vi "TDMSVisu.vi"(4 "error in (no error)":errorcluster caption="entrée d'erreur (pas d'erreur)", 7 "file path":path caption="chemin du fichier") -> (0 "error out":errorcluster caption="sortie d'erreur", 3 "file path out":path caption="chemin du fichier en sortie")   [LabVIEW 2017]
doc: "Ouvre le fichier .tdms spécifié dans l'entrée <B>chemin du fichier</B> et présente les données du fichier dans la boîte de dialogue TDMS - Afficheur de fichier."
uses:
  <vilib>/Utility/tdmsutil.llb/fileViewerConfigData.ctl
  <vilib>/Utility/error.llb/DialogType.ctl
  <vilib>/Utility/tdmsutil.llb/TDMSFileViewerLocalizedText.vi
  Instance           1 26Saved   TDMS - File Viewer .vi
panel:
  in  "Quit":bool caption="Quitter"
  in  "Properties / Values / Graph":T1(tab) caption="Propriétés / Valeurs / Graphe"
  in  "Properties":i32(listbox) caption="Propriétés"
  in  "Status":string caption="État"
  in  "Settings...":bool caption="Paramètres..."
  in  "Raw data values":i32(listbox) caption="Valeurs des données brutes"
  out "Waveform Graph":waveform(dbl)[](graph) caption="Graphe"
  in  "Help":bool caption="Aide"
  in  "File contents":string(tree) caption="Contenu du fichier"
  # "Affichage des valeurs 1..1000"
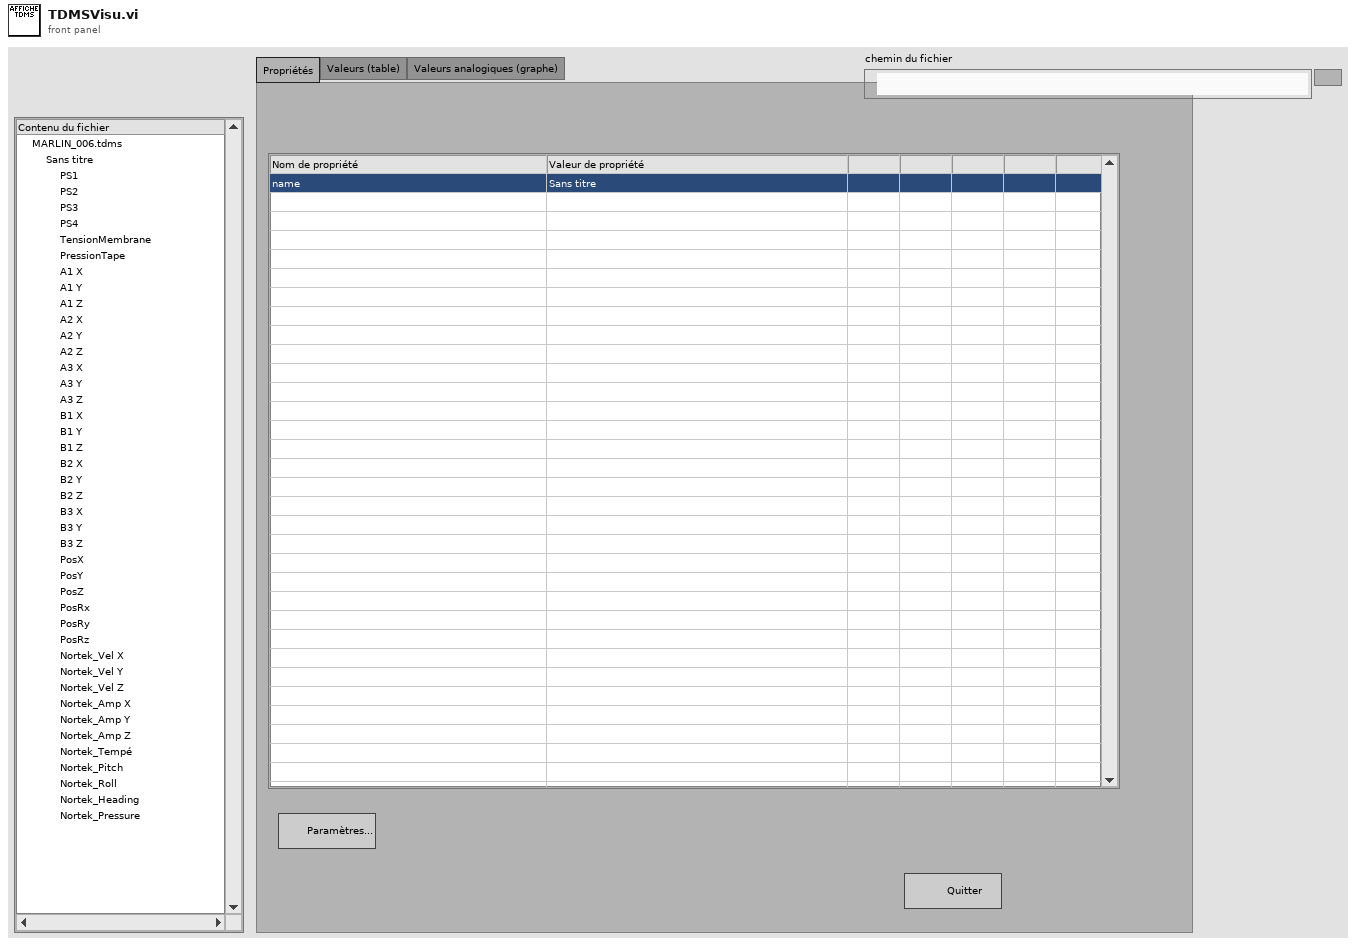
[diagram p1: front panel]
types:
  T1 = enum32{"Properties", "Values (table)", "Analog values (graph)"}
  T2 = enum16{"open", "open or create", "create or replace", "create", "open (read-only)"}
  T3 = typedef "fileViewerConfigData.ctl" = cluster{"Show all (table)":bool, "Show all (graph)":bool, "limit (table)":u64, "limit (graph)":u64, "no show":bool, "start (table)":u64, "start (graph)":u64}
  T4 = cluster{"Tree":refnum<vi>, "Tab Control":refnum<vi>, "property list":refnum<vi>, "raw data list":refnum<vi>, "Waveform Graph":refnum<vi>, "Ok":refnum<vi>, "Ok 2":refnum<vi>, "Ok 3":refnum<vi>, "Ok 4":refnum<vi>}
  T5 = typedef "DialogType.ctl" = u16
  T6 = typedef "LVRectTypeDef.ctl" = cluster{"Left":i16, "Top":i16, "Right":i16, "Bottom":i16}
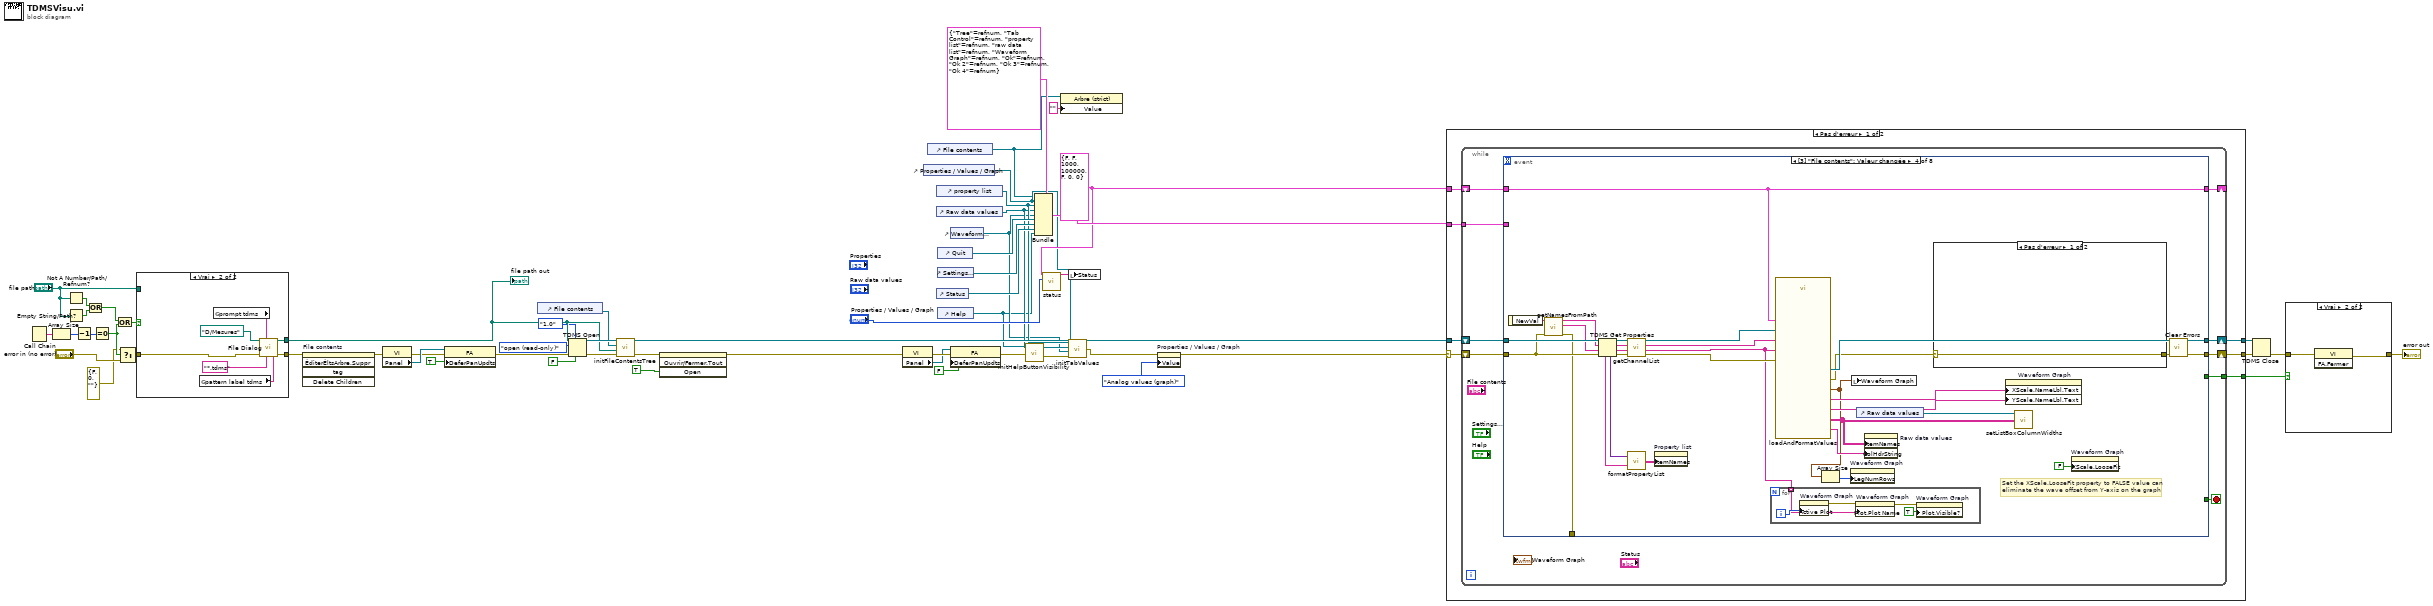
[diagram p0: block diagram]
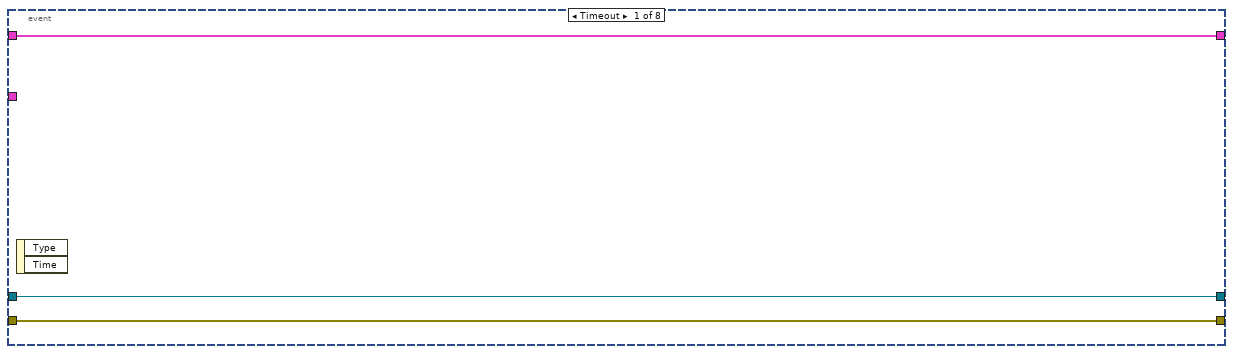
[diagram p3: hidden frame]
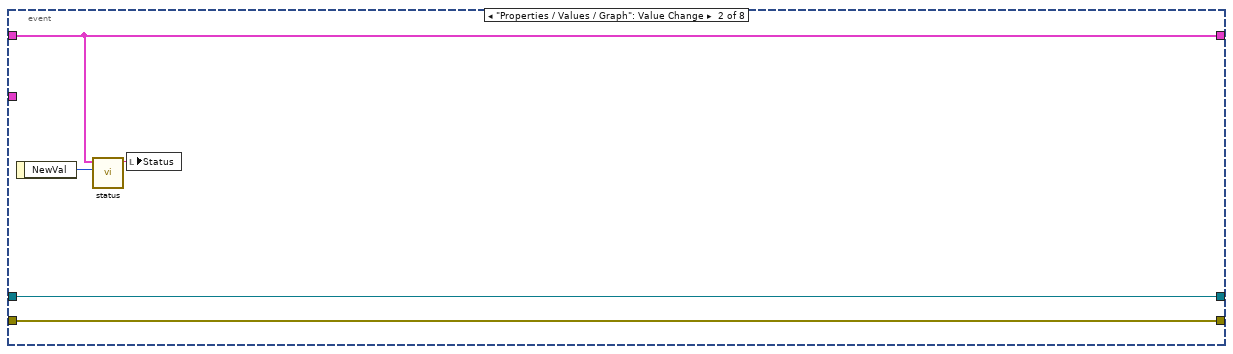
[diagram p4: hidden frame]
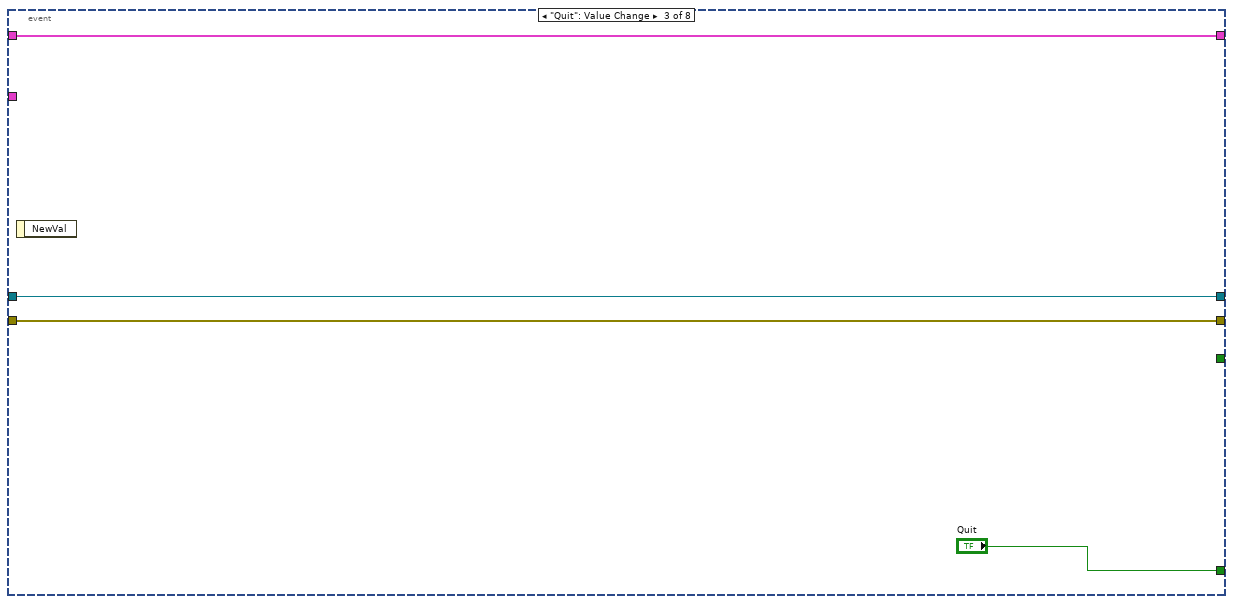
[diagram p5: hidden frame]
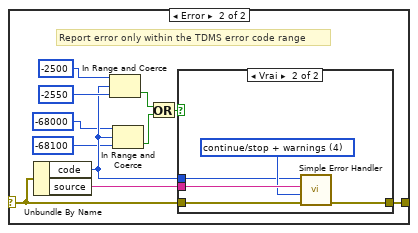
[diagram p6: hidden frame]
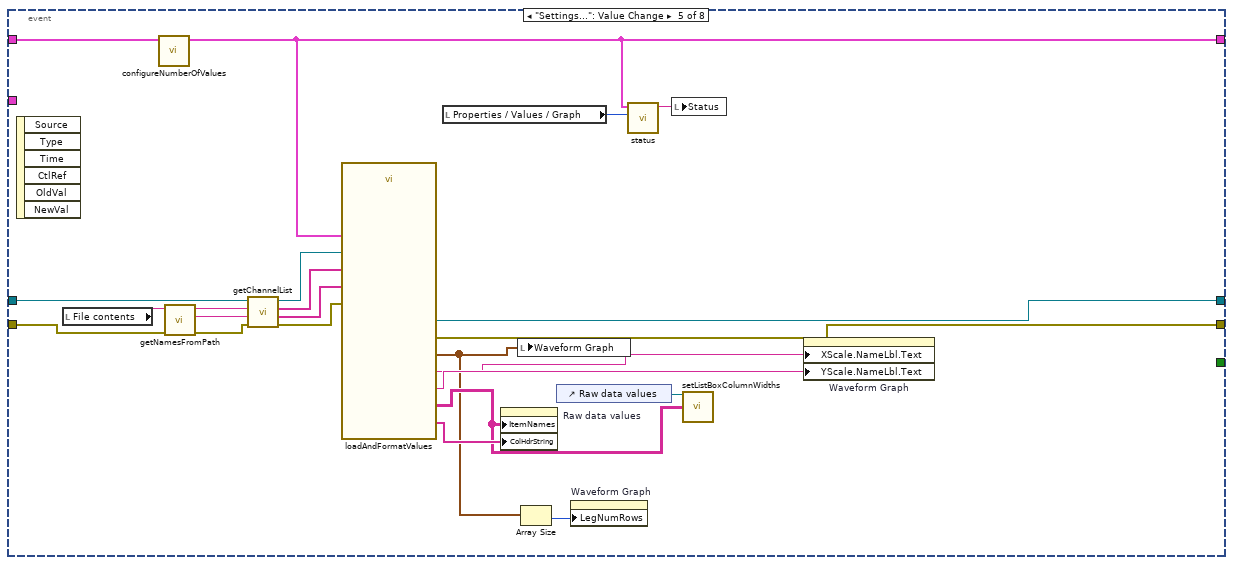
[diagram p8: hidden frame]
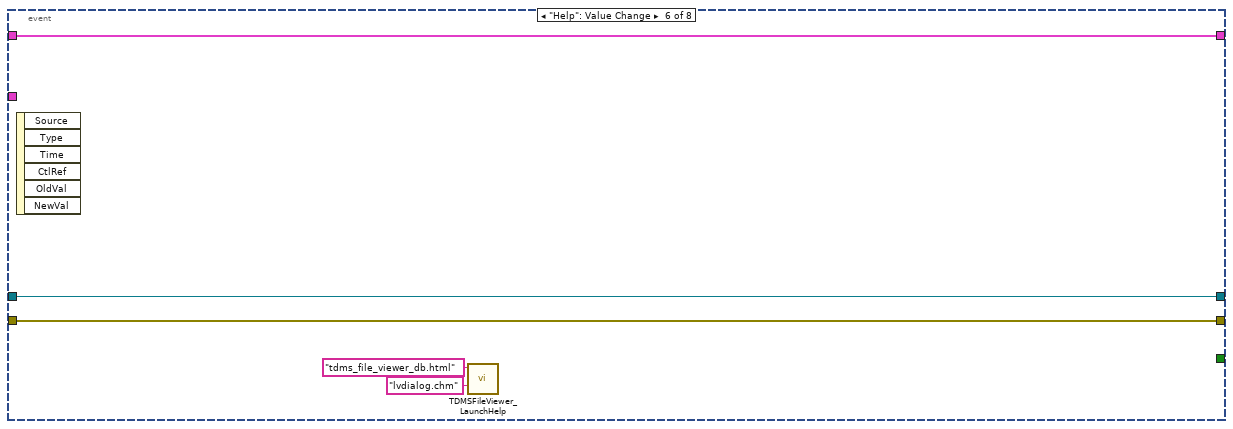
[diagram p9: hidden frame]
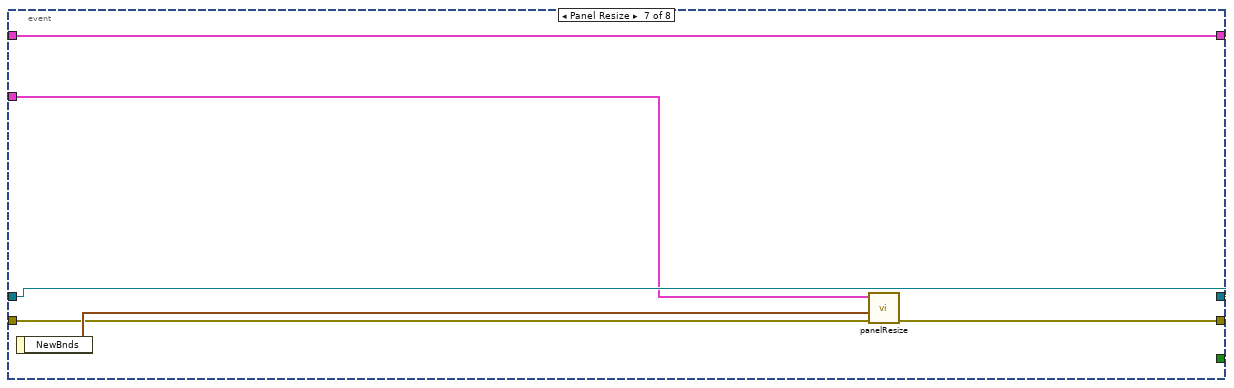
[diagram p10: hidden frame]
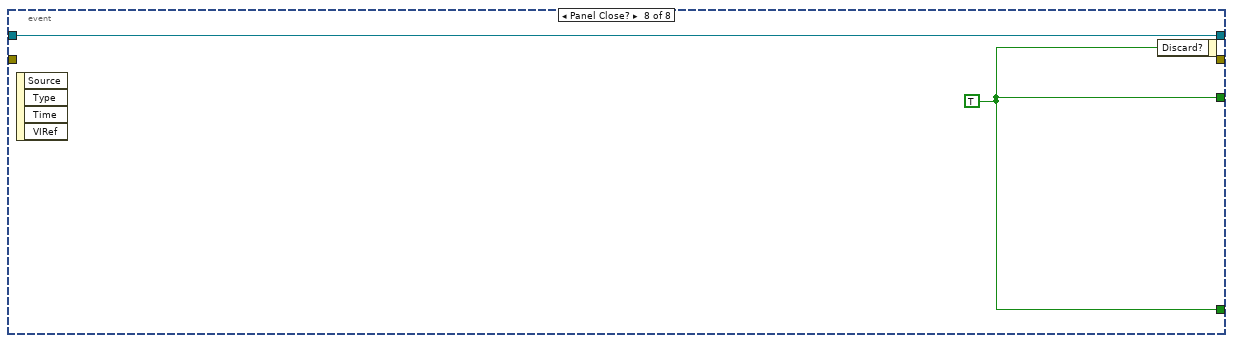
[diagram p11: hidden frame]
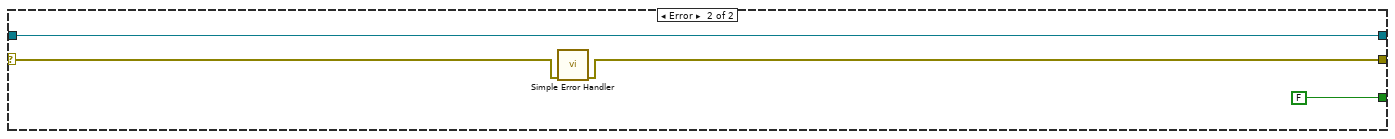
[diagram p12: hidden frame]
diagram:
  w24 = T3 {"Show all (table)"=FALSE, "Show all (graph)"=FALSE, "limit (table)"=1000, "limit (graph)"=100000, "no show"=FALSE, "start (table)"=0, "start (graph)"=0} ("TDMS File Viewer Configuration")
  n1 = Call Chain() -> (call chain=w39:string[])
  n2 = Array Size(array=w39) -> (size(s)=w37:i32)
  n3 = Not A Number/Path/Refnum?(number/path/refnum="file path") -> (NaN/Path/Refnum?=w41:bool)
  n4 = Empty String/Path?(string/path="file path") -> (empty?=w40:bool)
  n5 = Decrement(x=w37) -> (x-1=w36:i32)
  n6 = Or(x=w41, y=w40) -> (x .or. y?=w38:bool)
  n7 = Equal To 0?(x=w36) -> (x = 0?=w22:bool)
  n8 = Or(x=w38, y=w22) -> (x .or. y?=w35:bool)
  n9 = Select(t=errorcluster {"status"=FALSE, "code"=0, "source"=""}, s=w22, f="error in (no error)") -> (s? t:f=w21:errorcluster)
  n10 = case shown="Vrai" w35 {
    tunnel: [w59 w66] -> w28
    tunnel: "file path" -> [w59 _]
    tunnel: [w58 w64] -> w27
    tunnel: w21 -> [w58 w61]
    frame False {
    }
    frame True {
      n11 = global read "TDMSFileViewerLocalizedText.vi" "pattern label tdms"() -> (w62:string)
      n12 = global read "TDMSFileViewerLocalizedText.vi" "prompt tdms"() -> (w63:string)
      n13 = call "File Dialog"("start path"=path "D:/Mesures", "prompt"=w63, "error in"=w61, "pattern (all files)"="*.tdms", "pattern label"=w62) -> ("selected path"=w66:path, "error out"=w64:errorcluster)  [unwired: 2 in, 7 out]
    }
  }
  "file path out" <- w28
  n14 = invoke on="File contents" class="Tree (strict)" method="ÉditerÉltsArbre.Suppr"(error in=w27) -> (error out=w48:errorcluster)  [unwired: 4 in, 4 out]
  n15 = property class="VI"(error in=w48) -> (error out=w49:errorcluster, "Panel"=w50:refnum<vi>)  [unwired: 1 in, 1 out]
  n16 = property class="FA"(reference=w50, error in=w49, "DeferPanUpdts"=TRUE ("Defer Panel Updates")) -> (error out=w52:errorcluster)  [unwired: 1 out]
  n17 = control-ref of="File contents"() -> (w29:refnum<vi>)
  n18 = TDMS Open(6:FALSE ("disable buffering (T)"), 7:enum16{"1.0", "2.0"}."1.0" ("file format version (2.0)"), 8:w52, 10:T2."open (read-only)" ("operation"), 11:w28) -> (0:w57:errorcluster, 3:w56:refnum<k34>)  [unwired: 2 in]
  n19 = call <vilib>:"initFileContentsTree.vi"("error in (no error)"=w57, "file path"=w28, "Tree Refnum"=w29, "tdms file"=w56) -> ("error out"=w44:errorcluster, "tdms file out"=w55:refnum<k34>)  [unwired: 2 out]
  n20 = invoke on="File contents" class="Tree (strict)" method="Ouvrir/Fermer.Tout"(error in=w44, "Open"=TRUE ("Open?")) -> (error out=w3:errorcluster)  [unwired: 2 in, 3 out]
  n21 = property class="VI"(error in=w3) -> (error out=w46:errorcluster, "Panel"=w45:refnum<vi>)  [unwired: 1 in, 1 out]
  n22 = control-ref of="Properties / Values / Graph"() -> (w10:refnum<vi>)
  n23 = control-ref of="File contents"() -> (w9:refnum<vi>)
  n24 = control-ref of="property list"() -> (w13:refnum<vi>)
  n25 = control-ref of="Raw data values"() -> (w12:refnum<vi>)
  n26 = control-ref of="Status"() -> (w26:refnum<vi>)
  n27 = control-ref of="Quit"() -> (w33:refnum<vi>)
  n28 = control-ref of="Settings..."() -> (w31:refnum<vi>)
  n29 = control-ref of="Help"() -> (w5:refnum<vi>)
  n30 = control-ref of="Waveform Graph"() -> (w11:refnum<vi>)
  n31 = property class="FA"(reference=w45, error in=w46, "DeferPanUpdts"=FALSE ("Defer Panel Updates")) -> (error out=w7:errorcluster)  [unwired: 1 out]
  n32 = call <vilib>:"initHelpButtonVisibility.vi"("error in"=w7, "Help"=w5) -> ("error out"=w6:errorcluster)  [unwired: 9 in]
  n33 = Bundle(cluster=T4 {"Tree"=refnum, "Tab Control"=refnum, "property list"=refnum, "raw data list"=refnum, "Waveform Graph"=refnum, "Ok"=refnum, "Ok 2"=refnum, "Ok 3"=refnum, "Ok 4"=refnum} ("control refs"), "Tree"=w9, "Tab Control"=w10, "property list"=w13, "raw data list"=w12, "Waveform Graph"=w11, "Ok"=w33, "Ok 2"=w31, "Ok 3"=w26, "Ok 4"=w5) -> (w34:T4)
  n34 = call <vilib>:"status.vi"("tab sheet"="Properties / Values / Graph", "TDMS File Viewer Configuration"=w24) -> ("status"=w25:string)  [unwired: 5 out]
  n35 = property class="Arbre (strict)"(reference=w9, "Value"="") -> ()  [unwired: 1 in, 2 out]
  n36 = local write "Status"(w25) -> ()
  n37 = call <vilib>:"initTabValues.vi"("properties"=w13, "Values"=w12, "waveform"=w11, "error in"=w6, "Properties / Values / Graph"=w10) -> ("error out"=w2:errorcluster)
  n38 = property on="Properties / Values / Graph" class="Onglet (strict)"(error in=w2, "Value"=T1."Analog values (graph)" ("Properties / Values / Graph")) -> (error out=w1:errorcluster)  [unwired: 1 in, 1 out]
  n39 = case shown="Pas d'erreur" w1 {
    selector: w1 -> [w68 w186]
    tunnel: w55 -> [w73 w187]
    tunnel: [w72 w187] -> w54
    tunnel: [w71 w185] -> w53
    tunnel: w34 -> [w70 _]
    tunnel: w24 -> [w69 _]
    tunnel: [w67 FALSE] -> w18
    frame No Error {
      n40 = while {
        shift-right: [w80] -> w71
        shift-left: w68 -> [w81]
        shift-right: [w79] -> w72
        shift-left: w73 -> [w82]
        tunnel: w70 -> [w77]
        shift-right: [w75] -> _
        shift-left: w69 -> [w76]
        tunnel: [w74] -> w67
        stop <- w78 stop-if-true
        n41 = event shown="[3] \"File contents\": Valeur changée" {
          selector: _ -> [_ _ _ _ _ _ _ _]
          dyn-events: _ -> [_ _ _ _ _ _ _ _]
          timeout: _ -> [_ _ _ _ _ _ _ _]
          tunnel: w82 -> [w84 w89 w93 w124 w160 w174 w181 w183]
          tunnel: w81 -> [w85 w90 w92 w116 w167 w173 w178 _]
          tunnel: [w85 w90 w92 w112 w168 w173 w177 _] -> w80
          tunnel: [w84 w89 w93 w123 w169 w174 w181 w183] -> w79
          tunnel: [_ _ "Quit" _ _ _ _ w182] -> w78
          tunnel: [_ _ _ w115 _ _ _ _] -> _
          tunnel: w77 -> [_ _ _ _ _ _ w179 _]
          tunnel: w76 -> [w83 w86 w91 w105 w170 w175 w176 _]
          tunnel: [w83 w86 w91 w105 w150 w175 w176 _] -> w75
          tunnel: [_ _ _ _ _ _ _ w182] -> w74
          event Timeout {
            n42 = event-data() -> ()  [unwired: 3 out]
          }
          event "Properties / Values / Graph": Value Change {
            n43 = event-data() -> ("NewVal"=w88:T1)  [unwired: 1 out]
            n44 = call <vilib>:"status.vi"("tab sheet"=w88, "TDMS File Viewer Configuration"=w86) -> ("status"=w87:string)  [unwired: 5 out]
            n45 = local write "Status"(w87) -> ()
          }
          event "Quit": Value Change {
            n46 = event-data() -> ()  [unwired: 2 out]
          }
          event "File contents": Value Change {
            # "Set the XScale.LooseFit property to FALSE value can \neliminate the wave offset from Y-axis on the graph"
            n47 = event-data() -> ("NewVal"=w118:string)  [unwired: 1 out]
            n48 = call <vilib>:"getNamesFromPath.vi"("error in (no error)"=w116, "tree path"=w118) -> ("error out"=w115:errorcluster, "channel"=w121:string, "group"=w122:string)  [unwired: 3 out]
            n49 = TDMS Get Properties(8:w116, 9:w121, 10:w122, 11:w124) -> (0:w110:errorcluster, 1:w109:string, 2:w104:string, 3:w111:refnum<k34>, 4:w119:variant[], 6:w120:string[])  [unwired: 2 out]
            n50 = call <vilib>:"getChannelList.vi"("error in (no error)"=w110, "channel names"=w109, "group name"=w104, "tdms file"=w111) -> ("error out"=w101:errorcluster, "channel names out"=w95:string[], "group names out"=w102:string[], "tdms file out"=w103:refnum<k34>)
            n51 = call <vilib>:"formatPropertyList.vi"("property names"=w120, "property values"=w119) -> ("strings"=w117:string[][])
            n52 = property on="Property list" class="ListeMCol (strict)"("ItemNames"=w117) -> ()  [unwired: 2 in, 2 out]
            n53 = for {
              tunnel: w95 -> [w128] mode=indexing
              i -> [w129]
              n54 = property on="Waveform Graph" class="GraphWF (strict)"("Active Plot"=w129) -> (error out=w127:errorcluster)  [unwired: 2 in, 1 out]
              n55 = property on="Waveform Graph" class="GraphWF (strict)"(error in=w127, "Plot.Plot Name"=w128) -> (error out=w125:errorcluster)  [unwired: 1 in, 1 out]
              n56 = property on="Waveform Graph" class="GraphWF (strict)"(error in=w125, "Plot.Visible?"=TRUE ("Tracé.Visibles")) -> ()  [unwired: 1 in, 2 out]
            }
            n57 = call <vilib>:"loadAndFormatValues.vi"("error in (no error)"=w101, "configuration"=w105, "channel names"=w95, "group names"=w102, "tdms file"=w103) -> ("error out"=w100:errorcluster, "graph y names"=w107:string, "graph x names"=w106:string, "tdms file out"=w123:refnum<k34>, "waveform values"=w97:waveform(dbl)[], "table values"=w114:string[][], "table headers"=w108:string[])
            n58 = Array Size(array=w97) -> (size(s)=w96:i32)
            n59 = property on="Waveform Graph" class="GraphWF (strict)"("LegNumRows"=w96) -> ()  [unwired: 2 in, 2 out]
            n60 = local write "Waveform Graph"(w97) -> ()
            n61 = control-ref of="Raw data values"() -> (w113:refnum<vi>)
            n62 = property on="Raw data values" class="ListeMCol (strict)"("ItemNames"=w114, "ColHdrString"=w108) -> ()  [unwired: 2 in, 2 out]
            n63 = case shown="Pas d'erreur" w100 {
              selector: w100 -> [w130 w140]
              tunnel: [w130 w139] -> w99
              frame No Error {
              }
              frame Error {
                # "Report error only within the TDMS error code range"
                n64 = Unbundle By Name(w140) -> ("code"=w136:i32, "source"=w141:string)
                n65 = In Range and Coerce(upper limit=-2500, x=w136, lower limit=-2550 ("upper limit")) -> (In Range?=w133:bool)  [unwired: 1 out]
                n66 = In Range and Coerce(upper limit=-68000, x=w136, lower limit=-68100) -> (In Range?=w132:bool)  [unwired: 1 out]
                n67 = Or(x=w133, y=w132) -> (x .or. y?=w131:bool)
                n68 = case shown="Vrai" w131 {
                  tunnel: w141 -> [_ w147]
                  tunnel: w140 -> [w142 w146]
                  tunnel: [w142 w145] -> w139
                  tunnel: w136 -> [_ w143]
                  frame False {
                    # "Out of the range of TDMS\nerror code, we don't report\nthem."
                  }
                  frame True {
                    w144 = T5 4 items=["no dialog", "OK message", "continue or stop message", "OK message + warnings", "continue/stop + warnings"] ("type of dialog (OK msg:1)")
                    n69 = call <vilib>:"Simple Error Handler.vi"("error code (no error:0)"=w143, "error source (\" \")"=w147, "type of dialog (OK msg:1)"=w144, "error in (no error)"=w146) -> ("error out"=w145:errorcluster)  [unwired: 1 in, 4 out]
                  }
                }
              }
            }
            n70 = property on="Waveform Graph" class="GraphWF (strict)"("XScale.NameLbl.Text"=w106, "YScale.NameLbl.Text"=w107) -> ()  [unwired: 2 in, 2 out]
            n71 = call <vilib>:"setListBoxColumnWidths.vi"("table data"=w114, "MCListbox Refnum"=w113) -> ()  [unwired: 1 out]
            n72 = property on="Waveform Graph" class="GraphWF (strict)"("XScale.LooseFit"=FALSE ("X Scale.Loose Fit")) -> ()  [unwired: 2 in, 2 out]
            n73 = call <vilib>:"Clear Errors.vi"("error in (no error)"=w99) -> ("error out"=w112:errorcluster)  [unwired: 1 in, 5 out]
          }
          event "Settings...": Value Change {
            n74 = event-data() -> ()  [unwired: 7 out]
            n75 = local read "File contents"() -> (w161:string)
            n76 = call <vilib>:"configureNumberOfValues.vi"("TDMS File Viewer Configuration"=w170) -> ("TDMS File Viewer Configuration Out"=w150:T3)  [unwired: 10 out]
            n77 = call <vilib>:"getNamesFromPath.vi"("error in (no error)"=w167, "tree path"=w161) -> ("error out"=w159:errorcluster, "channel"=w157:string, "group"=w158:string)  [unwired: 3 out]
            n78 = call <vilib>:"getChannelList.vi"("error in (no error)"=w159, "channel names"=w157, "group name"=w158, "tdms file"=w160) -> ("error out"=w156:errorcluster, "channel names out"=w153:string[], "group names out"=w154:string[], "tdms file out"=w155:refnum<k34>)
            n79 = call <vilib>:"loadAndFormatValues.vi"("error in (no error)"=w156, "configuration"=w150, "channel names"=w153, "group names"=w154, "tdms file"=w155) -> ("error out"=w168:errorcluster, "graph y names"=w163:string, "graph x names"=w162:string, "tdms file out"=w169:refnum<k34>, "waveform values"=w148:waveform(dbl)[], "table values"=w164:string[][], "table headers"=w166:string[])
            n80 = local read "Properties / Values / Graph"() -> (w151:T1)
            n81 = property on="Raw data values" class="ListeMCol (strict)"("ItemNames"=w164, "ColHdrString"=w166) -> ()  [unwired: 2 in, 2 out]
            n82 = local write "Waveform Graph"(w148) -> ()
            n83 = Array Size(array=w148) -> (size(s)=w149:i32)
            n84 = control-ref of="Raw data values"() -> (w165:refnum<vi>)
            n85 = property on="Waveform Graph" class="GraphWF (strict)"("LegNumRows"=w149) -> ()  [unwired: 2 in, 2 out]
            n86 = call <vilib>:"status.vi"("tab sheet"=w151, "TDMS File Viewer Configuration"=w150) -> ("status"=w152:string)  [unwired: 5 out]
            n87 = local write "Status"(w152) -> ()
            n88 = call <vilib>:"setListBoxColumnWidths.vi"("table data"=w164, "MCListbox Refnum"=w165) -> ()  [unwired: 1 out]
            n89 = property on="Waveform Graph" class="GraphWF (strict)"("XScale.NameLbl.Text"=w162, "YScale.NameLbl.Text"=w163) -> ()  [unwired: 2 in, 2 out]
          }
          event "Help": Value Change {
            n90 = event-data() -> ()  [unwired: 7 out]
            n91 = call <vilib>:"TDMSFileViewer_LaunchHelp.vi"("CHM or HLP filename (lvdialog.chm)"="lvdialog.chm", "HTML filename"="tdms_file_viewer_db.html") -> ()  [unwired: 1 in, 5 out]
          }
          event Panel Resize {
            n92 = event-data() -> ("NewBnds"=w180:T6)  [unwired: 1 out]
            n93 = call <vilib>:"panelResize.vi"("error in (no error)"=w178, "NewBnds"=w180, "control refs"=w179) -> ("error out"=w177:errorcluster)  [unwired: 4 in]
          }
          event Panel Close? {
            w182 = TRUE
            n94 = event-data() -> ()  [unwired: 5 out]
            n95 = event-data("Discard?"=w182) -> ()  [unwired: 1 in, 1 out]
          }
        }
      }
    }
    frame Error {
      n96 = call <vilib>:"Simple Error Handler.vi"("error in (no error)"=w186) -> ("error out"=w185:errorcluster)  [unwired: 1 in, 7 out]
    }
  }
  n97 = TDMS Close(8:w53, 11:w54) -> (0:w17:errorcluster)  [unwired: 1 out]
  n98 = case shown="Vrai" w18 {
    tunnel: w17 -> [w188 w190]
    tunnel: [w188 w189] -> w16
    frame False {
    }
    frame True {
      n99 = invoke class="VI" method="FA.Fermer"(error in=w190) -> (error out=w189:errorcluster)  [unwired: 2 in, 2 out]
    }
  }
  "error out" <- w16
